vi "Create New Connection.vi"(8 "error in (no error)":errorcluster, 11 "Network Session Handler in":refnum<class "Network Session Handler.lvclass">) -> (0 "error out":errorcluster, 3 "Network Session Handler out":refnum<class "Network Session Handler.lvclass">, 4 "Next Timeout":i32)   [LabVIEW 2017, in "Network Interface.lvlib" / "Network Session Handler.lvclass"]
uses:
  <vilib>/gpm_packages/@cs/Network-sink/Source/Network Interface/Network Session Handler/Network Session Handler.lvclass
  <vilib>/gpm_packages/@cs/Network-sink/Source/Network Interface/Network Session Handler/Network Session Handler.lvclass/Network Session Handler.ctl
  <vilib>/gpm_packages/@cs/Network-sink/Source/Network Interface/IConnection/IConnection.lvclass
  <vilib>/gpm_packages/@cs/Network-sink/Source/Network Interface/Network Session Handler/Session Handler Message Names ENUM.ctl
  <vilib>/gpm_packages/@cs/Network-sink/Source/Network Interface/Message Queue/Message Queue.lvclass/Message Queue.ctl
  16bff32c-fbfc-4d6a-8be0-31aa02019e8b.vi
  <vilib>/gpm_packages/@cs/Network-sink/Source/Network Interface/Message Queue/Protected Enqueue.vi
  <vilib>/gpm_packages/@cs/Network-sink/Source/Network Interface/IConnectionFactory/IConnectionFactory.lvclass
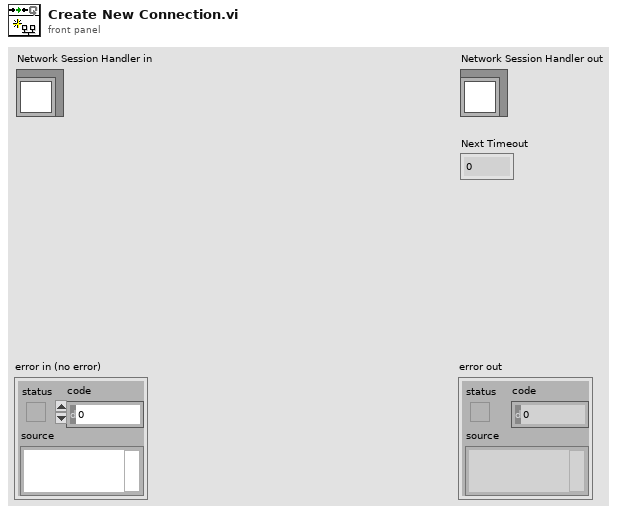
[diagram p1: front panel]
types:
  T1 = typedef "Network Interface.lvlib/Network Session Handler.lvclass/Session Handler Message Names ENUM.ctl" = enum16{"Transmit Message", "Stop", "Handler Shutdown", "Error"}
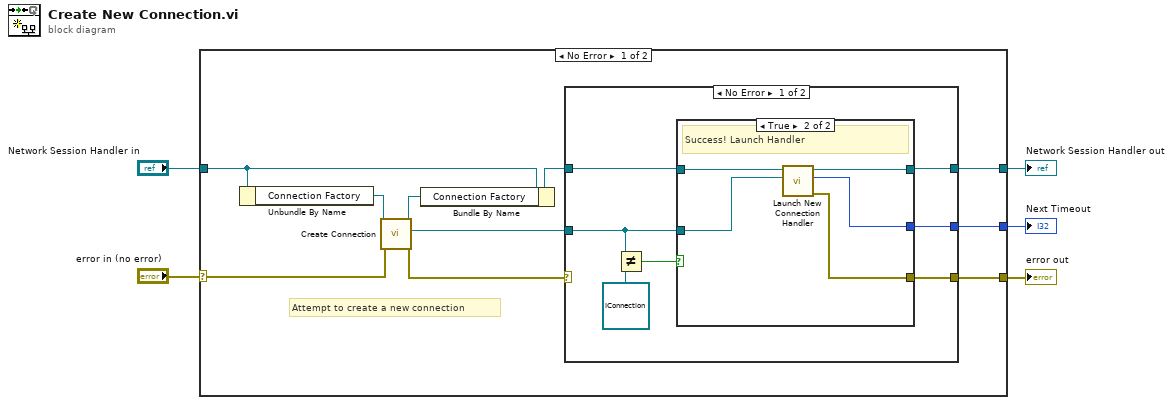
[diagram p0: block diagram]
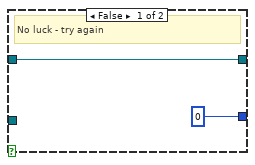
[diagram p2: hidden frame]
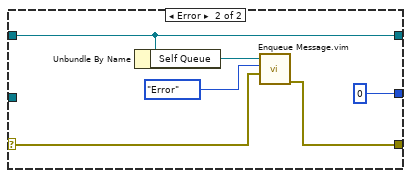
[diagram p3: hidden frame]
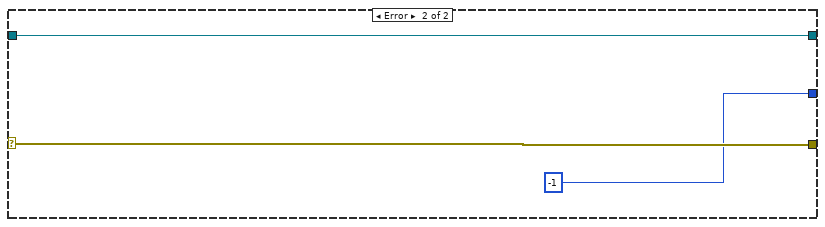
[diagram p4: hidden frame]
diagram:
  n1 = case shown="No Error" "error in (no error)" {
    selector: "error in (no error)" -> [w14 w38]
    tunnel: [w10 w38] -> w4
    tunnel: [w13 w37] -> w2
    tunnel: "Network Session Handler in" -> [w12 w37]
    tunnel: [w9 -1 ("Loop Timeout")] -> w1
    frame No Error {
      # "Attempt to create a new connection"
      n2 = Unbundle By Name(w12) -> ("Connection Factory"=w11:refnum<class "IConnectionFactory.lvclass">)
      n3 = call-dynamic "Create Connection.vi"("error in (no error)"=w14, "IConnectionFactory in"=w11) -> ("error out"=w15:errorcluster, "Connection"=w6:refnum<class "IConnection.lvclass">, "IConnectionFactory out"=w7:refnum<class "IConnectionFactory.lvclass">)  [unwired: 7 in]
      n4 = Bundle By Name(cluster=w12, "Connection Factory"=w7) -> (w8:refnum<class "Network Session Handler.lvclass">)
      n5 = case shown="No Error" w15 {
        selector: w15 -> [_ w32]
        tunnel: w6 -> [w18 _]
        tunnel: [w22 w35] -> w13
        tunnel: w8 -> [w21 w35]
        tunnel: [w20 w31] -> w10
        tunnel: [w19 0 ("Loop Timeout")] -> w9
        frame No Error {
          n6 = Not Equal?(x=w18, y=refnum<class "IConnection.lvclass"> refnum) -> (x != y?=w17:bool)
          n7 = case shown="True" w17 {
            tunnel: [_ w27] -> w20
            tunnel: w18 -> [_ w26]
            tunnel: [0 w25] -> w19
            tunnel: w21 -> [w23 w29]
            tunnel: [w23 w28] -> w22
            frame False {
              # "No luck - try again"
            }
            frame True {
              # "Success! Launch Handler"
              n8 = call <vilib>:"Launch New Connection Handler.vi"("Connection"=w26, "Network Session Handler in"=w29) -> ("error out"=w27:errorcluster, "Loop Timeout"=w25:i32, "Network Session Handler out"=w28:refnum<class "Network Session Handler.lvclass">)  [unwired: 7 in]
            }
          }
        }
        frame Error {
          n9 = Unbundle By Name(w35) -> ("Self Queue"=w34:refnum<class "Message Queue.lvclass">)
          n10 = call "Enqueue Message.vim"("Data"=w32, "Msg"=Session_Handler_Message_Names_ENUM."Error" ("Session Handler Messages"), "Message Queue in"=w34) -> ("error out"=w31:errorcluster)  [unwired: 7 in, 1 out]
        }
      }
    }
    frame Error {
    }
  }
  "error out" <- w4
  "Network Session Handler out" <- w2
  "Next Timeout" <- w1
